vi "CSM - Unregister Status Change.vi"(0 "CSM Name":string, 5 "Source CSM Name (* as Default)":string="*", 7 "Status":string, 9 "Response Message (\"*\" as Default)":string="*", 11 "Error In":errorcluster caption="error in (no error)") -> (4 "CSM Name (Dup)":string, 15 "error out":errorcluster)   [LabVIEW 2017, in "Communicable State Machine.lvlib"]
doc: "### CSM - Unregister Status Change.vi\n\nUnregister notifications of status changes from other CSM modules.\n\n-- <b>Controls</b> --\n- <b>CSM Name</b>: Name of the CSM module.\n- <b>Source CSM Name</b>: The CSM module generating the status. You can use \"*\" to denote all modules generating the same status.\n- <b>Status</b>: Status string.\n\n-- <b>Indicators</b> --\n- <b>CSM Name (dup)</b>: Returns <b>CSM Name</b>."
uses:
  Communicable State Machine.lvlib
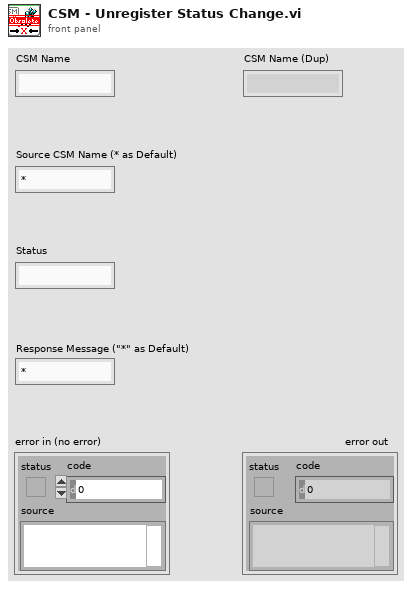
[diagram p1: front panel]
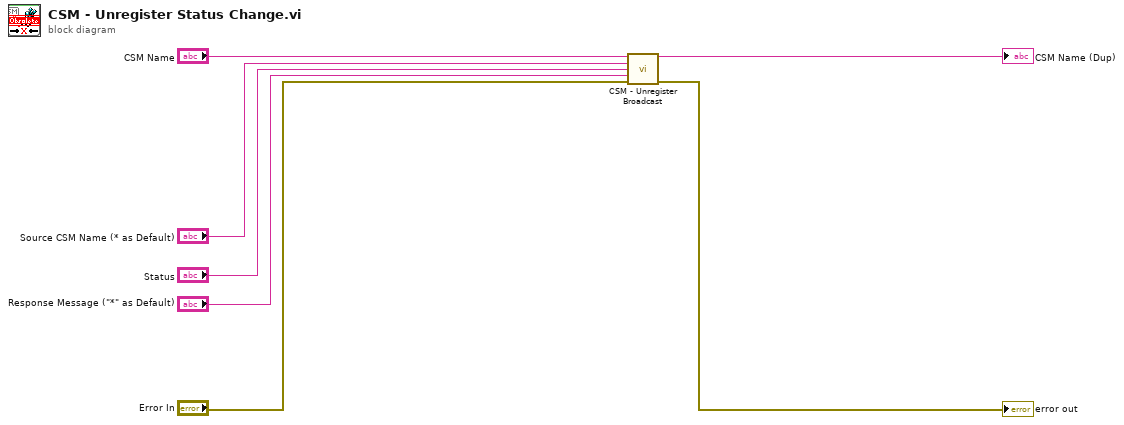
[diagram p0: block diagram]
diagram:
  n1 = call "CSM - Unregister Broadcast.vi"("CSM Name"="CSM Name", "Source CSM Name (* as Default)"="Source CSM Name (* as Default)", "Trigger"="Status", "API (\"*\" as Default)"="Response Message (\"*\" as Default)", "Error In"="Error In") -> ("CSM Name (Dup)"=→"CSM Name (Dup)":string, "error out"=→"error out":errorcluster)  [unwired: 9 in]
